vi "3458A Signalize Abort to Digitizing Process.vi"(8 "error in":errorcluster, 10 "send abort signal? (True)":bool=TRUE, 11 "session in":T1 {"channels"."Range [Vpk]" min=0.0}) -> (0 "error out (copy)":errorcluster, 3 "session out":T1 {"channels"."Range [Vpk]" min=0.0})   [LabVIEW 2018, in "3458A Virtual Digitizer.lvlib"]
doc: "This will signalize abort action to the digitizing process. The VI ignroes input error and will not generate any error."
uses:
  3458A Virtual Digitizer.lvlib
  3458A Digitizer Session.ctl
  3458A Virtual Channel Config.ctl
  Counter/Counter Session.ctl
  Counter/Counter Type.ctl
  AWG/AWG Session.ctl
  AWG/AWG Type.ctl
  3458A Sync Mode.ctl
  3458A Idn Mode.ctl
  3458A Digitizing Low Levels/Configure/Sampling Mode.ctl
  3458A Digitizing Process Options.ctl
  3458A Data Packet.ctl
  3458A Aux Record Data.ctl
  3458A Digitizing Low Levels/Configure/Level Setup.ctl
  3458A Digitizing Low Levels/Configure/First Sample Trigger.ctl
  3458A Aperture Selection Mode.ctl
  Counter/Counter.lvlib
  AWG/AWG.lvlib
  3458A Digitizing Low Levels/3458A Digitizing Low Levels.lvlib
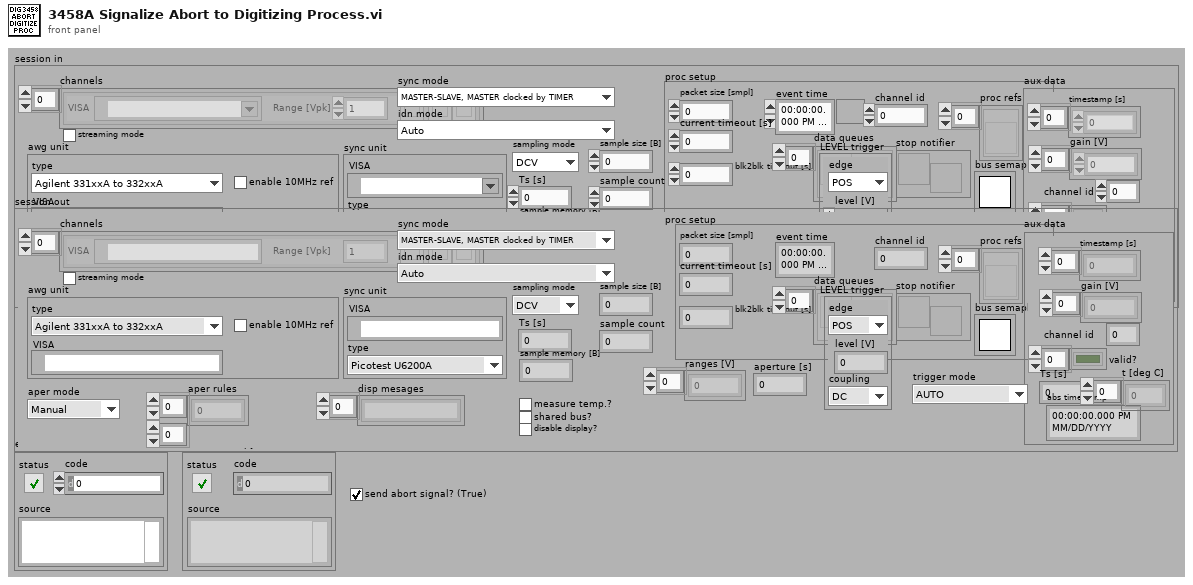
[diagram p1: front panel]
types:
  T1 = typedef "3458A Virtual Digitizer.lvlib/3458A Digitizer Session.ctl" = cluster{"channels":T2[], "sync unit":T3, "awg unit":T5, "sync mode":T7, "streaming mode":bool, "idn mode":T8, "sampling mode":T9, "Ts [s]":dbl, "sample memory [B]":i32, "proc setup":T10, "sample size [B]":i32, "sample count":i32, "aux data":T12, "ranges [V]":dbl[], "aperture [s]":dbl, "LEVEL trigger":T13, "trigger mode":T14, "measure temp.?":bool, "disp mesages":string[], "shared bus?":bool, "disable display?":bool, "aper mode":T15, "aper rules":dbl[][]}
  T2 = typedef "3458A Virtual Digitizer.lvlib/3458A Virtual Channel Config.ctl" = cluster{"VISA":refnum<visa-resource-name>, "Range [Vpk]":dbl, "btn clr":bool, "btn up":bool, "btn down":bool}
  T3 = typedef "Counter.lvlib/Counter Session.ctl" = cluster{"VISA":refnum<visa-resource-name>, "type":T4}
  T4 = typedef "Counter.lvlib/Counter Type.ctl" = enum16{"Picotest U6200A", "dummy"}
  T5 = typedef "AWG.lvlib/AWG Session.ctl" = cluster{"type":T6, "VISA":refnum<visa-resource-name>, "enable 10MHz ref":bool}
  T6 = typedef "AWG.lvlib/AWG Type.ctl" = enum16{"Agilent 331xxA to 332xxA", "Agilent 335xxA to 336xxA", "Tektronix AFG3101C", "dummy"}
  T7 = typedef "3458A Virtual Digitizer.lvlib/3458A Sync Mode.ctl" = enum16{"MASTER-SLAVE, MASTER clocked by TIMER", "MASTER-SLAVE, MASTER clocked by AWG", "ALL clocked by AWG", "MASTER-SLAVE, ALL clocked by TIMER", "ALL clocked by AWG with DFLL"}
  T8 = typedef "3458A Virtual Digitizer.lvlib/3458A Idn Mode.ctl" = enum16{"Auto", "Sequential (chn A, chn B, ...)", "From calibration string"}
  T9 = typedef "3458A Virtual Digitizer.lvlib/3458A Digitizing Low Levels.lvlib/Sampling Mode.ctl" = enum16{"DCV", "DSDC", "DSAC"}
  T10 = typedef "3458A Virtual Digitizer.lvlib/3458A Digitizing Process Options.ctl" = cluster{"channel id":i32, "packet size [smpl]":i32, "current timeout [s]":dbl, "blk2blk timeout [s]":dbl, "event time":timestamp, "stop notifier":refnum<notifier>, "data queues":refnum<queue>[], "proc refs":refnum<vi>[], "bus semaphore":T11}
  T11 = typedef "Semaphore RefNum" = refnum<k1>
  T12 = typedef "3458A Virtual Digitizer.lvlib/3458A Aux Record Data.ctl" = cluster{"channel id":i32, "valid?":bool[], "gain [V]":dbl[], "timestamp [s]":dbl[], "Ts [s]":dbl, "abs timestamp":timestamp, "t [deg C]":dbl[]}
  T13 = typedef "3458A Virtual Digitizer.lvlib/3458A Digitizing Low Levels.lvlib/Level Setup.ctl" = cluster{"edge":enum16{"POS", "NEG"}, "level [V]":dbl, "coupling":enum16{"DC", "AC"}}
  T14 = typedef "3458A Virtual Digitizer.lvlib/3458A Digitizing Low Levels.lvlib/First Sample Trigger.ctl" = enum16{"AUTO", "EXT", "SYN", "SGL", "HOLD", "LEVEL"}
  T15 = typedef "3458A Virtual Digitizer.lvlib/3458A Aperture Selection Mode.ctl" = enum16{"Manual", "Maximum", "Table"}
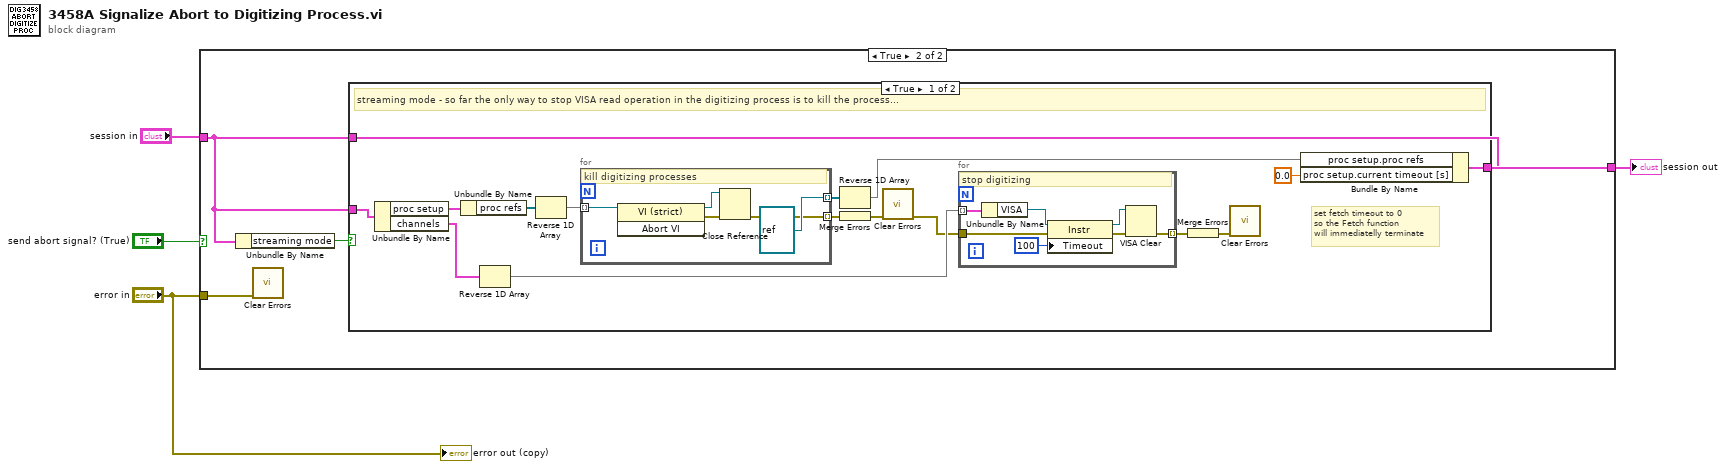
[diagram p0: block diagram]
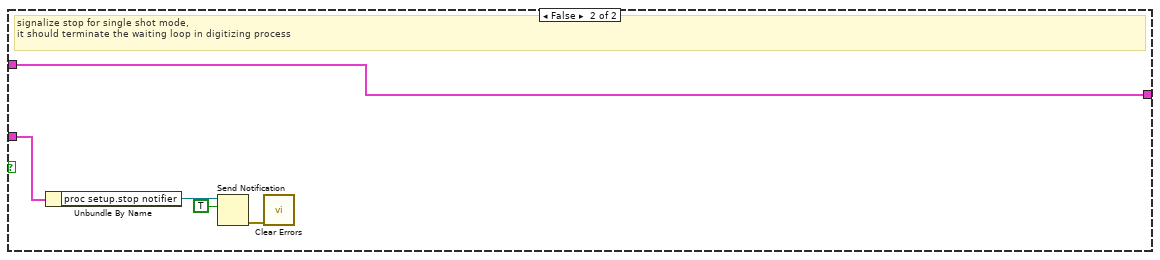
[diagram p3: hidden frame]
diagram:
  n1 = case shown="True" "send abort signal? (True)" {
    tunnel: "session in" -> [w5 w7]
    tunnel: "error in" -> [_ w9]
    tunnel: [w5 w6] -> w2
    frame False {
    }
    frame True {
      n2 = Unbundle By Name(w7) -> ("streaming mode"=w8:bool)
      n3 = call <vilib>:"Clear Errors.vi"("error in (no error)"=w9) -> ()  [unwired: 5 in, 2 out]
      n4 = case shown="True" w8 {
        tunnel: w7 -> [w25 w39]
        tunnel: w7 -> [w12 w38]
        tunnel: [w19 w38] -> w6
        frame True {
          # "set fetch timeout to 0\nso the Fetch function\nwill immediatelly terminate"
          # "streaming mode - so far the only way to stop VISA read operation in the digitizing process is to kill the process..."
          n5 = Unbundle By Name(w25) -> ("proc setup"=w24:T10, "channels"=w17:T2[])
          n6 = Unbundle By Name(w24) -> ("proc refs"=w23:refnum<vi>[])
          n7 = Reverse 1D Array(array=w17) -> (reversed array=w16:T2[])
          n8 = Reverse 1D Array(array=w23) -> (reversed array=w22:refnum<vi>[])
          n9 = for {
            tunnel: w22 -> [w37] mode=indexing
            tunnel: [w33] -> w21 mode=indexing
            tunnel: [refnum<vi> refnum ("new element/subarray")] -> w13 mode=indexing
            # "kill digitizing processes"
            n10 = invoke class="VI (strict)" method="Abort VI"(reference=w37) -> (reference out=w34:refnum<vi>, error out=w35:errorcluster)  [unwired: 2 in, 1 out]
            n11 = Close Reference(reference=w34, error in (no error)=w35) -> (error out=w33:errorcluster)
          }
          n12 = Reverse 1D Array(array=w13) -> (reversed array=w11:refnum<vi>[])
          n13 = Merge Errors(w21) -> (w20:errorcluster)
          n14 = call <vilib>:"Clear Errors.vi"("error in (no error)"=w20) -> ("error out"=w10:errorcluster)  [unwired: 5 in, 1 out]
          n15 = for {
            tunnel: w16 -> [w32] mode=indexing
            tunnel: [w31] -> w14 mode=indexing
            tunnel: w10 -> [w30]
            # "stop digitizing"
            n16 = Unbundle By Name(w32) -> ("VISA"=w28:refnum<visa-resource-name>)
            n17 = property class="Instr"(reference=w28, error in=w30, "Timeout"=u32 100 ("General Settings:Timeout Value")) -> (reference out=w27:refnum<visa-resource-name>, error out=w29:errorcluster)
            n18 = VISA Clear(VISA resource name=w27, error in (no error)=w29) -> (error out=w31:errorcluster)  [unwired: 1 out]
          }
          n19 = Merge Errors(w14) -> (w15:errorcluster)
          n20 = call <vilib>:"Clear Errors.vi"("error in (no error)"=w15) -> ()  [unwired: 5 in, 2 out]
          n21 = Bundle By Name(cluster=w12, "proc setup.proc refs"=w11, "proc setup.current timeout [s]"=0.0) -> (w19:T1)
        }
        frame False {
          # "signalize stop for single shot mode,\nit should terminate the waiting loop in digitizing process"
          n22 = Unbundle By Name(w39) -> ("proc setup.stop notifier"=w42:refnum<notifier>)
          n23 = Send Notification(notification=TRUE, notifier=w42) -> (error out=w40:errorcluster)  [unwired: 1 in, 1 out]
          n24 = call <vilib>:"Clear Errors.vi"("error in (no error)"=w40) -> ()  [unwired: 5 in, 2 out]
        }
      }
    }
  }
  "session out" <- w2
  "error out (copy)" <- "error in"
